vi "SLL Check the filename for windows format v1.vi"(11 "File Name":string) -> (3 "File Name OK?":bool)   [LabVIEW 2013]
doc: "Checks for the file name for windows format. If the file name is not comply with the windows format, the boolean will be FALSE.\n\nCopyright © 2006, Soliton Technologies. All rights reserved."
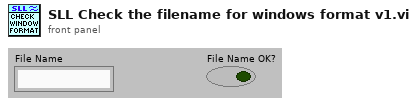
[diagram p1: front panel]
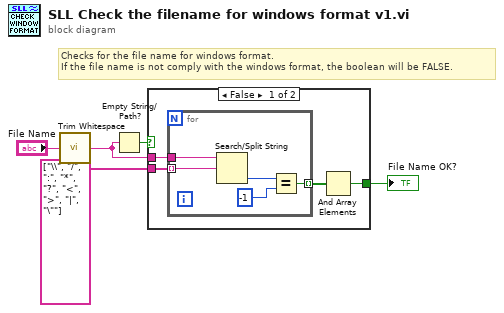
[diagram p0: block diagram]
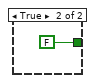
[diagram p2: hidden frame]
diagram:
  # "Checks for the file name for windows format. \nIf the file name is not comply with the windows format, the boolean will be FALSE."
  n1 = call <vilib>:"Trim Whitespace.vi"("string"="File Name") -> ("trimmed string"=w2:string)  [unwired: 1 in]
  n2 = Empty String/Path?(string/path=w2) -> (empty?=w1:bool)
  n3 = case shown="False" w1 {
    tunnel: [w9 FALSE] -> w5
    tunnel: string[] ["\\", "/", ":", "*", "?", "<", ">", "|", "\""] ("Array Constant") -> [w8 _]
    tunnel: w2 -> [w6 _]
    frame False {
      n4 = for {
        tunnel: w8 -> [w14] mode=indexing
        tunnel: [w11] -> w7 mode=indexing
        tunnel: w6 -> [w10]
        n5 = Search/Split String(string=w10, search string/char (-)=w14) -> (offset of match=w13:i32)  [unwired: 1 in, 2 out]
        n6 = Equal?(x=w13, y=-1) -> (x = y?=w11:bool)
      }
      n7 = And Array Elements(Boolean array=w7) -> (logical AND=w9:bool)
    }
    frame True {
    }
  }
  "File Name OK?" <- w5
